vi "CurrentPositionGet.vi"(3 "error in (no error)":errorcluster, 5 "VISA resource name":refnum<visa-resource-name>) -> (0 "error out":errorcluster, 1 "Position":cluster{"Numeric":dbl, "Units":string}, 2 "VISA resource name out":refnum<visa-resource-name>)   [LabVIEW 2017, in "Spectral Products CM110.lvlib"]
uses:
  Spectral Products CM110.lvlib
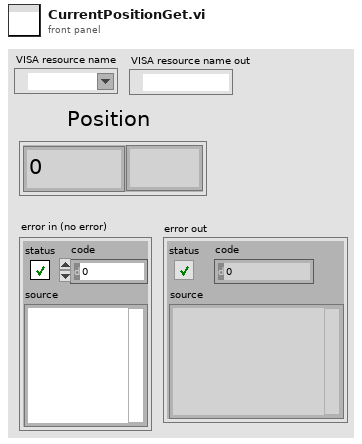
[diagram p1: front panel]
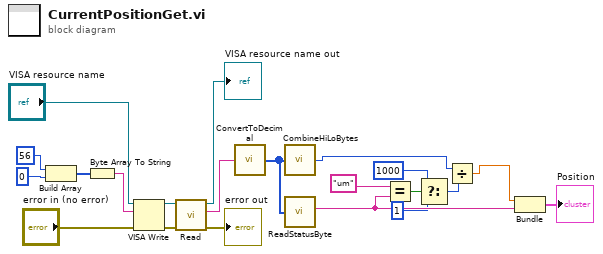
[diagram p0: block diagram]
diagram:
  n1 = Build Array(u8 56, u8 0) -> (w12:u8[])
  n2 = Byte Array To String(unsigned byte array=w12) -> (string=w10:string)
  n3 = VISA Write(VISA resource name="VISA resource name", write buffer=w10, error in (no error)="error in (no error)") -> (VISA resource name out=w20:refnum<visa-resource-name>, error out=w21:errorcluster)  [unwired: 1 out]
  n4 = call "Read.vi"("error in (no error)"=w21, "VISA Refnum in"=w20) -> ("error out"=→"error out":errorcluster, "read buffer"=w15:string, "VISA Refnum out"=→"VISA resource name out":refnum<visa-resource-name>)  [unwired: 6 in, 1 out]
  n5 = call "ConvertToDecimal.vi"("read buffer"=w15) -> ("unsigned byte array"=w14:u8[])
  n6 = call "CombineHiLoBytes.vi"("unsigned byte array"=w14) -> ("Numeric"=w2:u16)
  n7 = call "ReadStatusByte.vi"("unsigned byte array"=w14) -> ("Units"=w8:string)  [unwired: 4 in, 5 out]
  n8 = Equal?(x="um", y=w8) -> (x = y?=w6:bool)
  n9 = Select(t=i16 1000, s=w6, f=i16 1) -> (s? t:f=w3:i16)
  n10 = Divide(x=w2, y=w3) -> (x/y=w1:dbl)
  n11 = Bundle(w1, "Units"=w8) -> (→"Position":cluster{dbl, "Units":string})  [unwired: 1 in]
